vi "2-ReadAllFiles.vi"(8 "error in (no error)":errorcluster, 11 "AllControls IN":T1) -> (0 "error out":errorcluster, 3 "AllControls Out":T1)   [LabVIEW 2017]
uses:
  Ctrls/AllControls.ctl
  <vilib>/Utility/miscctls.llb/LVRowAndColumnTypeDef.ctl
  Ctrls/Position Config.ctl
  Ctrls/TesterInfo.ctl
  Ctrls/HD Config.ctl
  <vilib>/Utility/file.llb/Read Delimited Spreadsheet (string).vi
  ComVIS/Files/Ini/ReadIniFiles_ByVarient.vi
  <vilib>/regexp/Match Regular Expression.xnode
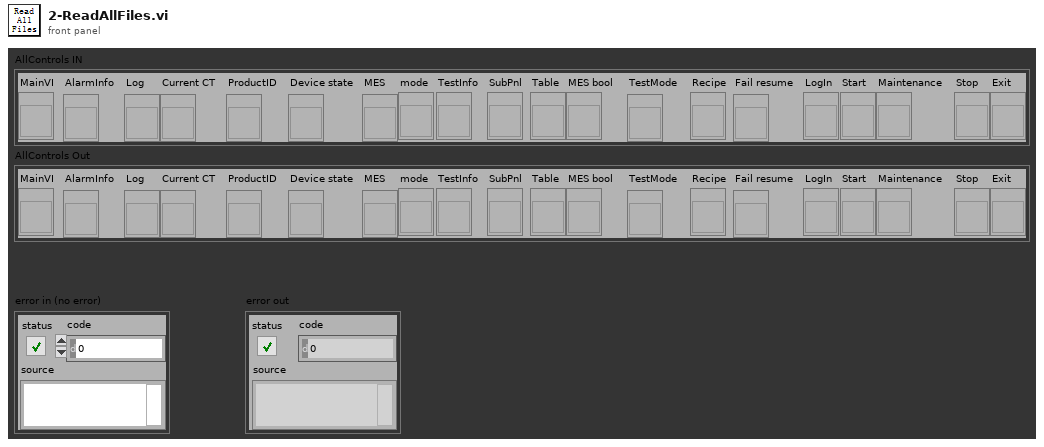
[diagram p1: front panel]
types:
  T1 = typedef "AllControls.ctl" = cluster{"MainVI":refnum<vi>, "AlarmInfo":refnum<vi>, "Log":refnum<vi>, "Current CT":refnum<vi>, "ProductID":refnum<vi>, "Device state":refnum<vi>, "MES":refnum<vi>, "mode":refnum<vi>, "TestInfo":refnum<vi>, "SubPnl":refnum<vi>, "Table":refnum<vi>, "MES bool":refnum<vi>, "TestMode":refnum<vi>, "Recipe":refnum<vi>, "Fail resume":refnum<vi>, "LogIn":refnum<vi>, "Start":refnum<vi>, "Maintenance":refnum<vi>, "Stop":refnum<vi>, "Exit":refnum<vi>}
  T2 = typedef "HD Config.ctl" = cluster{" PC":cluster{"PC Address":u8[], "PC Port":i32}, "FCO":cluster{"COM":refnum<visa-resource-name>, "Baudrate":u32}, "DC Power ":cluster{"COM":refnum<visa-resource-name>, "Baudrate":u32}, "PW3336":cluster{"COM":refnum<visa-resource-name>, "Baudrate":u32}, "Lefoo":cluster{"COM":refnum<visa-resource-name>, "Baudrate":u32}, "Tempt&Hum":cluster{"COM":refnum<visa-resource-name>, "Baudrate":u32}, "DIPC":cluster{"COM":refnum<visa-resource-name>}, "Daemon":cluster{"IP Address":string, "Port":u16, "Retry":u16}, "URAT":cluster{"COM":refnum<visa-resource-name>, "Baudrate":u32}, "Fail_resume_mode":bool, "GRR":bool}
  T3 = typedef "TesterInfo.ctl" = cluster{"Station Name":string, "Station Code":string, "ES NO.":string, "Tester ID":string, "PassMark Revision":string, "Rig ID":string, "Deamon_vision":string, "Project Name":string, "FFTesterPath":path, "Enable_User":bool, "Mode":enum16{"682"}, "MES":bool}
  T4 = typedef "Position Config.ctl" = cluster{"OrificeSize_12.7":i32, "OrificeSize_13":i32, "OrificeSize_30":i32, "OrificeSize_16":i32}
  T5 = typedef "LVRowAndColumnTypeDef.ctl" = cluster{"Row":i32, "Column":i32}
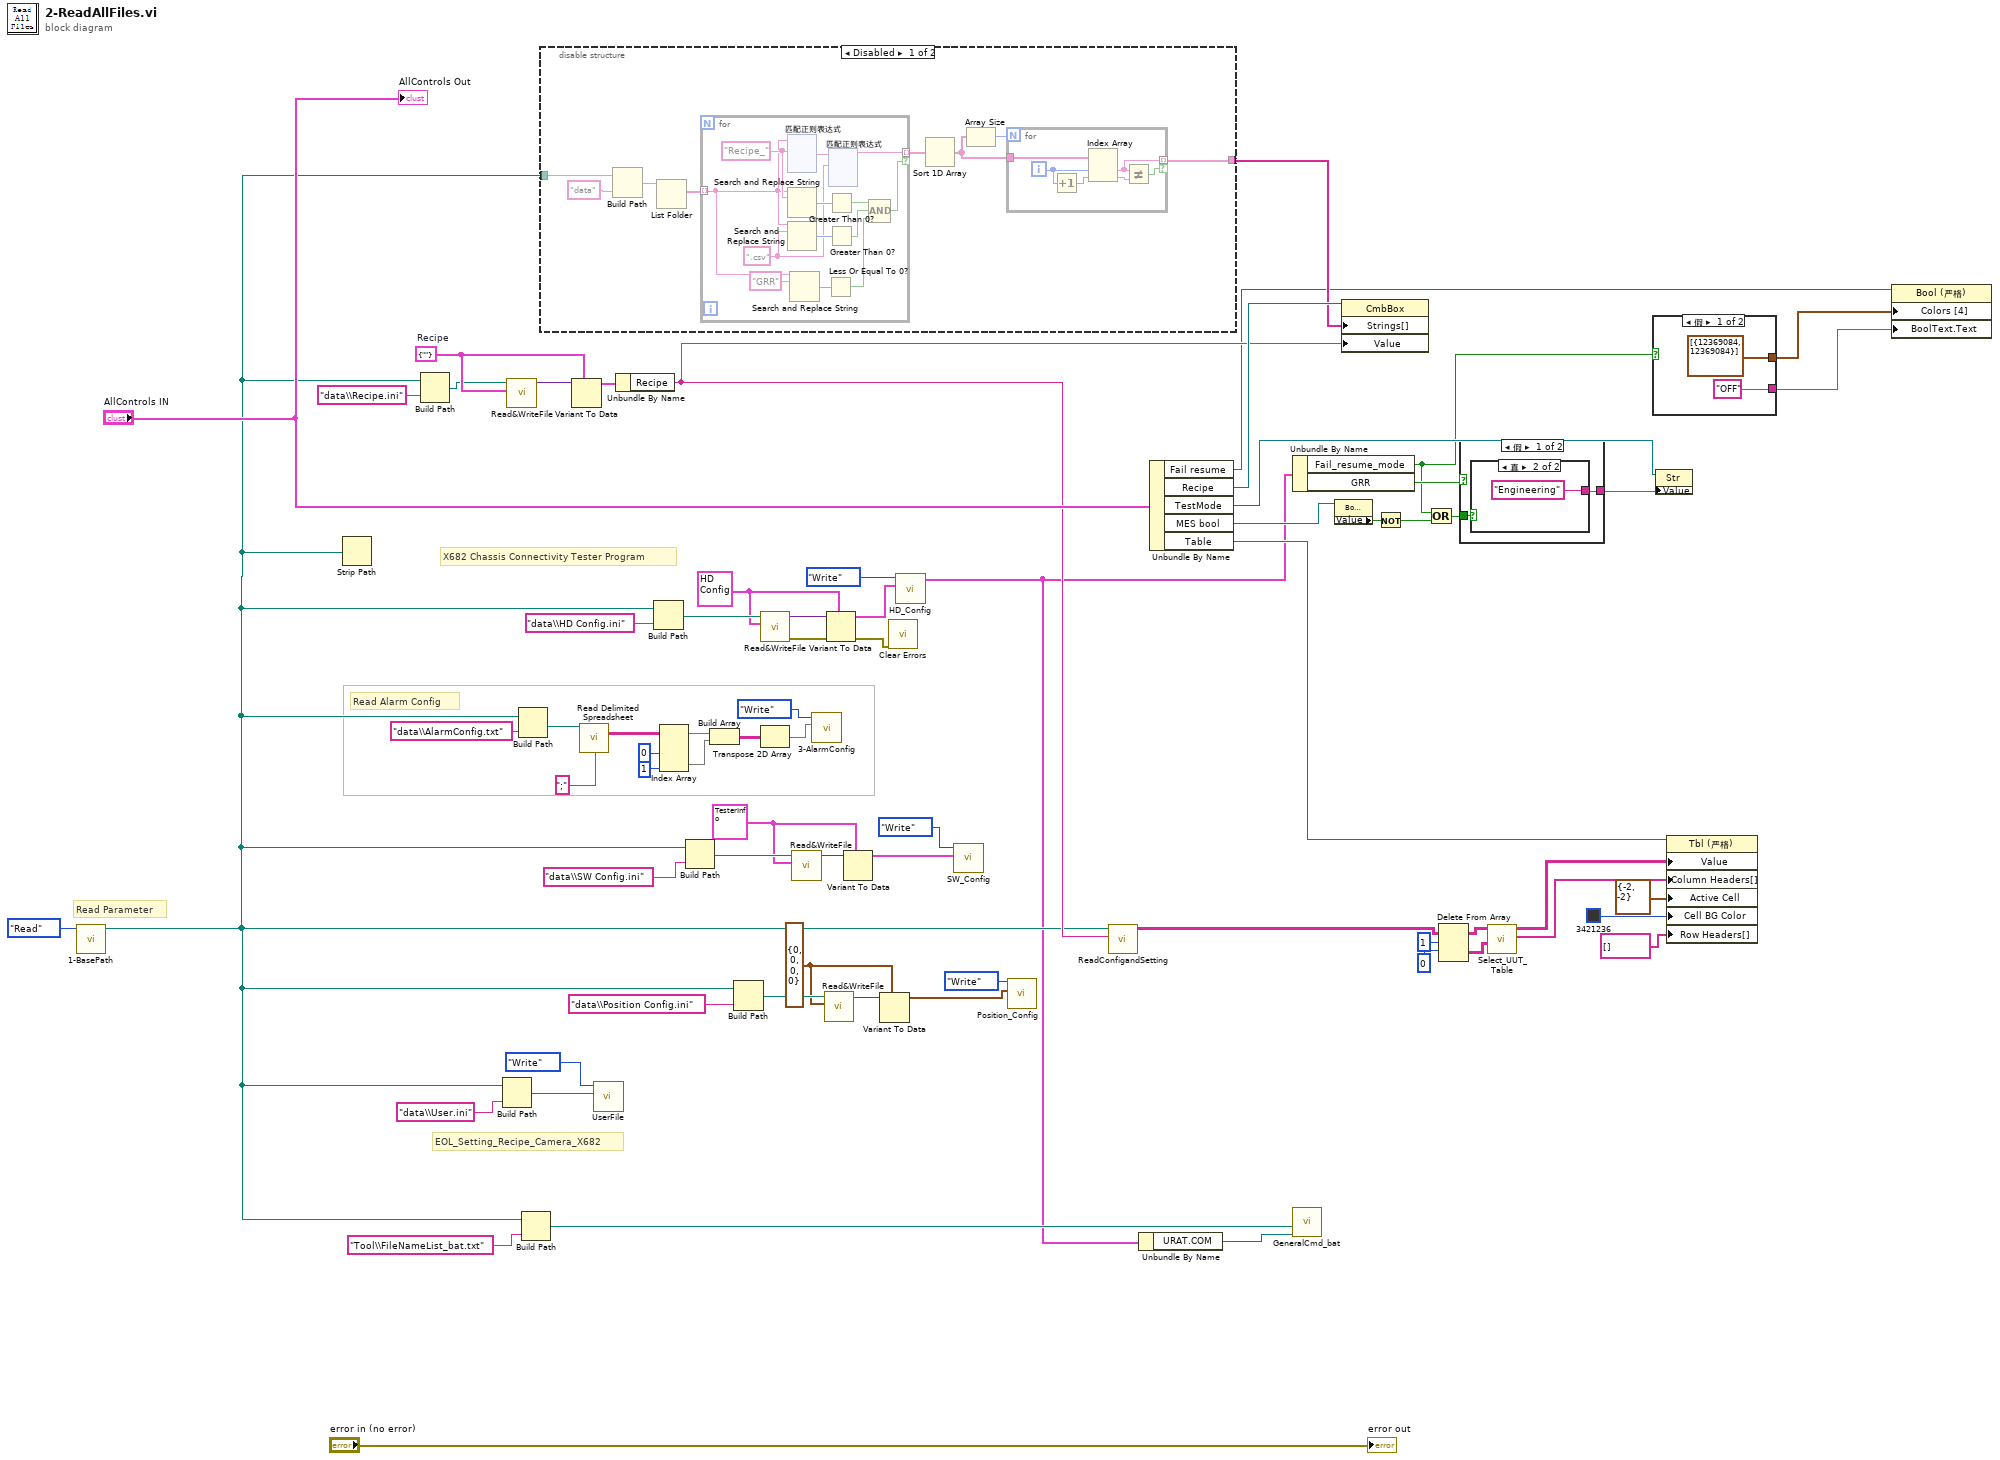
[diagram p0: block diagram]
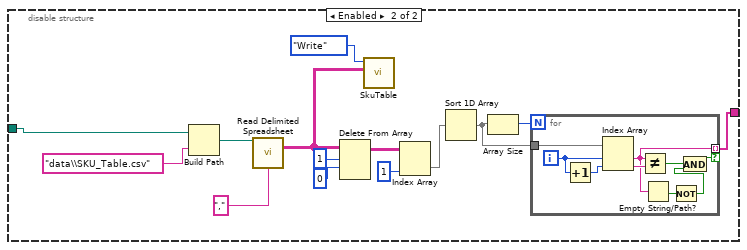
[diagram p2: hidden frame]
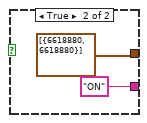
[diagram p3: hidden frame]
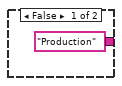
[diagram p4: hidden frame]
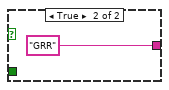
[diagram p5: hidden frame]
diagram:
  w15 = cluster{"Recipe":string} {"Recipe"=""}  # Recipe
  w26 = T2 {" PC"={"PC Address"=[], "PC Port"=0}, "FCO"={"COM"="", "Baudrate"=0}, "DC Power "={"COM"="", "Baudrate"=0}, "PW3336"={"COM"="", "Baudrate"=0}, "Lefoo"={"COM"="", "Baudrate"=0}, "Tempt&Hum"={"COM"="", "Baudrate"=0}, "DIPC"={"COM"=""}, "Daemon"={"IP Address"="", "Port"=0, "Retry"=0}, "URAT"={"COM"="", "Baudrate"=0}, "Fail_resume_mode"=FALSE, "GRR"=FALSE} ("HD Config")
  w27 = T3 {"Station Name"="", "Station Code"="", "ES NO."="", "Tester ID"="", "PassMark Revision"="", "Rig ID"="", "Deamon_vision"="", "Project Name"="", "FFTesterPath"=path "", "Enable_User"=FALSE, "Mode"=enum."682", "MES"=FALSE} ("TesterInfo")
  w30 = T4 {"OrificeSize_12.7"=0, "OrificeSize_13"=0, "OrificeSize_30"=0, "OrificeSize_16"=0} ("Position Config")
  # "X682 Chassis Connectivity Tester Program"
  # "EOL_Setting_Recipe_Camera_X682"
  # "Read Alarm Config"
  # "Read Parameter"
  n1 = call "1-BasePath.vi"("Step"=enum16{"Initial", "Write", "Read"}."Read") -> ("Path Out"=w4:path)  [unwired: 9 in, 1 out]
  n2 = Strip Path(path=w4) -> ()  [unwired: 2 out]
  n3 = Build Path(base path=w4, name or relative path="data\\Recipe.ini") -> (appended path=w12:path)
  n4 = Build Path(base path=w4, name or relative path="data\\User.ini") -> (appended path=w48:path)
  n5 = call-poly "Read&WriteFile.vi"("Varient"=w15, "path"=w12) -> ("DataOut"=w16:variant)  [unwired: 8 in, 1 out]
  n6 = Build Path(base path=w4, name or relative path="data\\AlarmConfig.txt") -> (appended path=w63:path)
  n7 = Build Path(base path=w4, name or relative path="Tool\\FileNameList_bat.txt") -> (appended path=w3:path)
  n8 = disable-structure shown="Disabled" {
    disable-tunnel: [w74 w330] -> w17
    disable-tunnel: w4 -> [w73 w337]
    frame Disabled {
      n9 = Build Path(base path=w73, name or relative path="data") -> (appended path=w79:path)
      n10 = List Folder(path=w79) -> (filenames=w78:string[])  [unwired: 3 in, 3 out]
      n11 = for {
        tunnel: w78 -> [w90] mode=indexing
        tunnel: [w91] -> w77 mode=indexing if=w97
        w92 = ".csv" ("搜索字符串")
        w94 = "Recipe_" ("搜索字符串")
        n12 = xnode "匹配正则表达式"("输入字符串"=w90, "正则表达式"=w94) -> ("匹配之后"=w93:string)  [unwired: 4 in, 4 out]
        n13 = Search and Replace String(input string=w90, search string=w94) -> (number of replacements=w99:i32)  [unwired: 6 in, 3 out]
        n14 = Search and Replace String(input string=w90, search string=w92) -> (number of replacements=w96:i32)  [unwired: 6 in, 3 out]
        n15 = Search and Replace String(input string=w90, search string="GRR" ("搜索字符串")) -> (number of replacements=w88:i32)  [unwired: 6 in, 3 out]
        n16 = Less Or Equal To 0?(x=w88) -> (x <= 0?=w87:bool)
        n17 = Greater Than 0?(x=w99) -> (x > 0?=w98:bool)
        n18 = Greater Than 0?(x=w96) -> (x > 0?=w95:bool)
        n19 = xnode "匹配正则表达式"("输入字符串"=w93, "正则表达式"=w92) -> ("匹配之前"=w91:string)  [unwired: 4 in, 4 out]
        n20 = Compound Arithmetic op=AND ("复合运算")(w98, w95, w87) -> (w97:bool)
      }
      n21 = Sort 1D Array(array=w77) -> (sorted array=w75:string[])
      n22 = Array Size(array=w75) -> (size(s)=w76:i32)
      n23 = for {
        N: w76 -> [_]
        tunnel: w75 -> [w86]
        tunnel: [w82] -> w74 mode=indexing if=w85
        i -> [w84]
        n24 = Increment(x=w84) -> (x+1=w83:i32)
        n25 = Index Array(array=w86, index #1=w84, index #2=w83) -> (element #1=w82:string, element #2=w81:string)
        n26 = Not Equal?(x=w82, y=w81) -> (x != y?=w85:bool)
      }
    }
    frame Enabled {
      n27 = Build Path(base path=w337, name or relative path="data\\SKU_Table.csv") -> (appended path=w341:path)
      n28 = call-poly <vilib>:"Read Delimited Spreadsheet.vi"("file path (dialog if empty)"=w341, "delimiter (\\t)"="," ("delimiter (\\t)")) -> ("all rows"=w336:string[][])  [unwired: 8 in, 5 out]
      n29 = Delete From Array(array=w336, length=1 ("长度"), index (row)=0 ("索引 (行)")) -> (array with subset deleted=w333:string[][])  [unwired: 1 in, 1 out]
      n30 = call "SkuTable.vi"("Tabledata in"=w336, "Step"=enum16{"Initial", "Write", "Read"}."Write") -> ()  [unwired: 8 in, 2 out]
      n31 = Index Array(array=w333, index (col)=1 ("禁用的索引 (列)")) -> (element=w328:string[])  [unwired: 1 in]
      n32 = Sort 1D Array(array=w328) -> (sorted array=w329:string[])
      n33 = Array Size(array=w329) -> (size(s)=w331:i32)
      n34 = for {
        N: w331 -> [_]
        tunnel: w329 -> [w350]
        tunnel: [w345] -> w330 mode=indexing if=w343
        i -> [w348]
        n35 = Increment(x=w348) -> (x+1=w347:i32)
        n36 = Index Array(array=w350, index #1=w348, index #2=w347) -> (element #1=w345:string, element #2=w346:string)
        n37 = Not Equal?(x=w345, y=w346) -> (x != y?=w349:bool)
        n38 = Empty String/Path?(string/path=w345) -> (empty?=w344:bool)
        n39 = Not(x=w344) -> (.not. x?=w342:bool)
        n40 = And(x=w349, y=w342) -> (x .and. y?=w343:bool)
      }
    }
  }
  n41 = Variant To Data(type=w15, Variant=w16) -> (data=w14:cluster{"Recipe":string})  [unwired: 1 in, 1 out]
  n42 = call-poly <vilib>:"Read Delimited Spreadsheet.vi"("file path (dialog if empty)"=w63, "delimiter (\\t)"=";" ("delimiter (\\t)")) -> ("all rows"=w60:string[][])  [unwired: 8 in, 5 out]
  n43 = call "UserFile.vi"("UserPath in"=w48, "Step"=enum16{"Initial", "Write", "Read"}."Write") -> ()  [unwired: 8 in, 2 out]
  n44 = Unbundle By Name(w14) -> ("Recipe"=w11:string)
  n45 = Build Path(base path=w4, name or relative path="data\\HD Config.ini") -> (appended path=w68:path)
  n46 = Index Array(array=w60, index (col) #1=0 ("disabled index (col)"), index (col) #2=1 ("index (col)")) -> (element #1=w59:string[], element #2=w55:string[])  [unwired: 2 in]
  n47 = Build Path(base path=w4, name or relative path="data\\SW Config.ini") -> (appended path=w52:path)
  n48 = Build Array(w59, w55) -> (w56:string[][])
  n49 = Build Path(base path=w4, name or relative path="data\\Position Config.ini") -> (appended path=w33:path)
  n50 = call-poly "Read&WriteFile.vi"("Varient"=w26, "path"=w68) -> ("error out"=w66:errorcluster, "DataOut"=w67:variant)  [unwired: 8 in]
  n51 = Transpose 2D Array(2D array=w56) -> (transposed array=w54:string[][])
  n52 = call-poly "Read&WriteFile.vi"("Varient"=w27, "path"=w52) -> ("DataOut"=w50:variant)  [unwired: 8 in, 1 out]
  n53 = call "3-AlarmConfig.vi"("AlarmConfig In"=w54, "Step"=enum16{"Initial", "Write", "Read"}."Write") -> ()  [unwired: 8 in, 2 out]
  n54 = call-poly "Read&WriteFile.vi"("Varient"=w30, "path"=w33) -> ("DataOut"=w31:variant)  [unwired: 8 in, 1 out]
  n55 = Variant To Data(error in=w66, type=w26, Variant=w67) -> (data=w46:T2, error out=w65:errorcluster)
  n56 = Variant To Data(type=w27, Variant=w50) -> (data=w45:T3)  [unwired: 1 in, 1 out]
  n57 = Variant To Data(type=w30, Variant=w31) -> (data=w29:T4)  [unwired: 1 in, 1 out]
  n58 = call <vilib>:"Clear Errors.vi"("error in (no error)"=w65) -> ()  [unwired: 5 in, 2 out]
  n59 = call "HD_Config.vi"("HD Config in"=w46, "Step"=enum16{"Initial", "Write", "Read"}."Write") -> ("HD Config out"=w1:T2)  [unwired: 8 in, 1 out]
  n60 = call "SW_Config.vi"("SW Config In"=w45, "Step"=enum16{"Initial", "Write", "Read"}."Write") -> ()  [unwired: 8 in, 2 out]
  n61 = call "Position_Config.vi"("Position Config"=w29, "Step"=enum16{"Initial", "Write", "Read"}."Write") -> ()  [unwired: 8 in, 2 out]
  n62 = call "ReadConfigandSetting.vi"("Recipe"=w11, "Path Out"=w4) -> ("TableData"=w37:string[][])  [unwired: 7 in, 2 out]
  n63 = Unbundle By Name(w1) -> ("URAT.COM"=w2:refnum<visa-resource-name>)
  n64 = Unbundle By Name("AllControls IN") -> ("Fail resume"=w8:refnum<vi>, "Recipe"=w18:refnum<vi>, "TestMode"=w23:refnum<vi>, "MES bool"=w24:refnum<vi>, "Table"=w39:refnum<vi>)
  n65 = Unbundle By Name(w1) -> ("Fail_resume_mode"=w9:bool, "GRR"=w25:bool)
  n66 = call "GeneralCmd_bat.vi"("COM"=w2, "fileList_bat"=w3) -> ()  [unwired: 9 in, 1 out]
  n67 = property class="Bool (严格)"(reference=w24) -> ("Value"=w21:bool)  [unwired: 1 in, 2 out]
  n68 = property class="CmbBox"(reference=w18, "Strings[]"=w17, "Value"=w11) -> ()  [unwired: 1 in, 2 out]
  n69 = Not(x=w21) -> (.not. x?=w19:bool)
  n70 = Or(x=w9, y=w19) -> (x .or. y?=w20:bool)
  n71 = Delete From Array(array=w37, length=1 ("长度"), index (row)=0 ("索引 (行)")) -> (deleted portion=w35:string[][], array with subset deleted=w38:string[][])  [unwired: 1 in]
  n72 = case shown="假" w25 {
    tunnel: w20 -> [w352 _]
    tunnel: [w351 "GRR"] -> w22
    frame False {
      n73 = case shown="真" w352 {
        tunnel: ["Production" "Engineering"] -> w351
        frame False {
        }
        frame True {
        }
      }
    }
    frame True {
    }
  }
  n74 = call "Select_UUT_Table.vi"("all Title"=w35, "all Table"=w38) -> ("Title"=w36:string[], "Table"=w10:string[][])  [unwired: 8 in]
  n75 = case shown="假" w9 {
    tunnel: [cluster{u32, u32}[] [{12369084, 12369084}] cluster{u32, u32}[] [{6618880, 6618880}]] -> w7
    tunnel: ["OFF" "ON"] -> w6
    frame False {
    }
    frame True {
    }
  }
  n76 = property class="Str"(reference=w23, "Value"=w22) -> ()  [unwired: 1 in, 2 out]
  n77 = property class="Tbl (严格)"(reference=w39, "Value"=w10, "Column Headers[]"=w36, "Active Cell"=T5 {"Row"=-2, "Column"=-2} ("活动单元格:活动单元格"), "Cell BG Color"=u32 3421236, "Row Headers[]"=string[] [] ("Row Header Strings[]")) -> ()  [unwired: 1 in, 2 out]
  n78 = property on="属性节点" class="Bool (严格)"(reference=w8, "Colors [4]"=w7, "BoolText.Text"=w6) -> ()  [unwired: 1 in, 2 out]
  "AllControls Out" <- "AllControls IN"
  "error out" <- "error in (no error)"
